vi "Add_to_speed_calib_file.vi"(2 "Desired Velocity":dbl format="%.2f", 3 "Max Velocity":dbl format="%.2f", 4 "New Row":dbl[](array[numeric]) format="%.2f", 6 "Rig Name":string, 7 "Mode":enum16{"Add Row", "Get Error Value"}(ring)) -> (0 "Tweaked Demand":dbl format="%.4f", 1 "Calib Tweak %":dbl format="%.4f")   [LabVIEW 2015]
uses:
  Anemometry/Anemometry Sub Vis/File/Setup_Filetype.ctl
  Anemometry/Anemometry Sub Vis/Controls/In_Range.ctl
panel:
  out "Array":dbl[][](array[numeric]) format="%.4f"
  out "Channel Values":string[][](array[string])
  # "Dem Vel       Calib Tweak   Meas Vel"
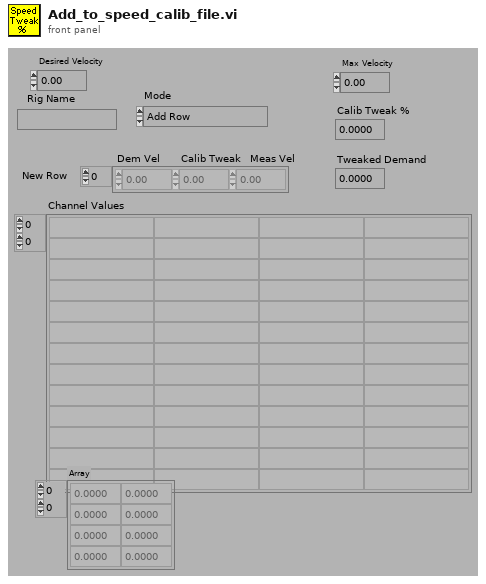
[diagram p1: front panel]
types:
  T1 = typedef "Setup_Filetype.ctl" = enum16{"Measurement Setups", "Calibration Setups", "General", "Results File Plotter Setups", "Speed Calib Tweaks"}
  T2 = typedef "In_Range.ctl" = enum16{"%", "±", "% & ±"}
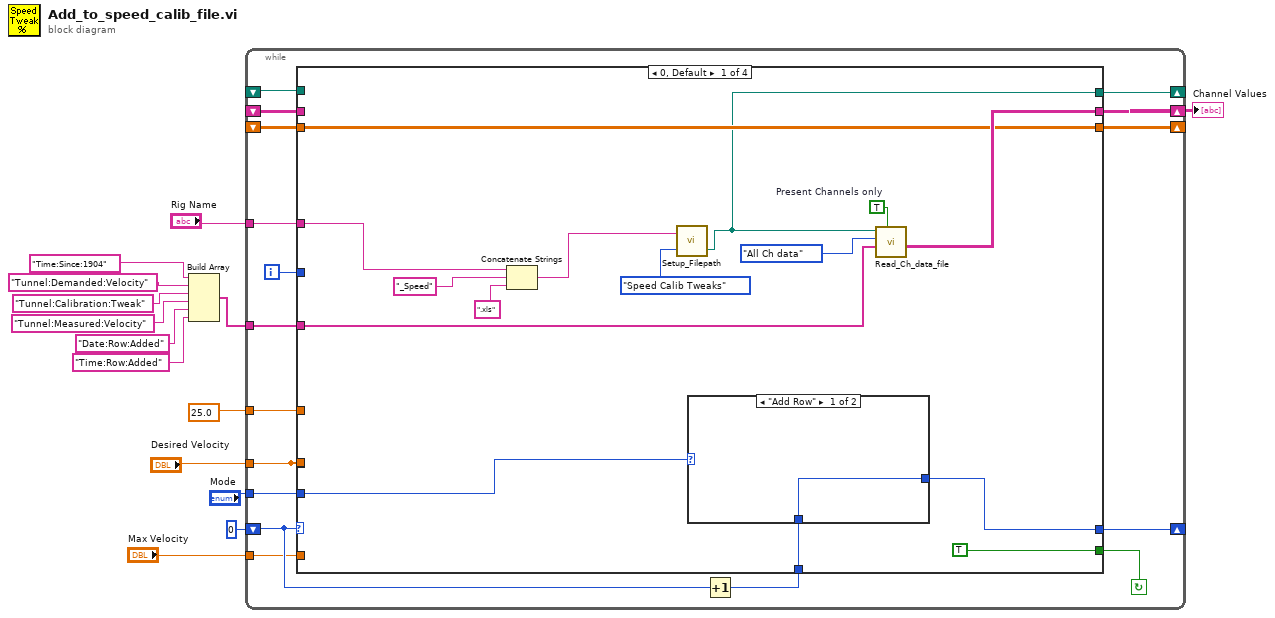
[diagram p0: block diagram]
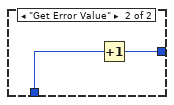
[diagram p2: hidden frame]
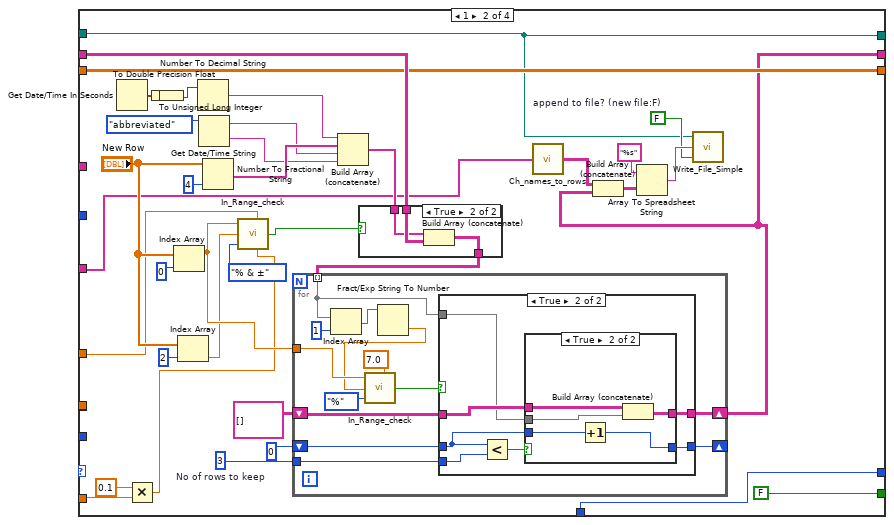
[diagram p3: hidden frame]
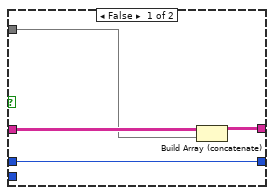
[diagram p5: hidden frame]
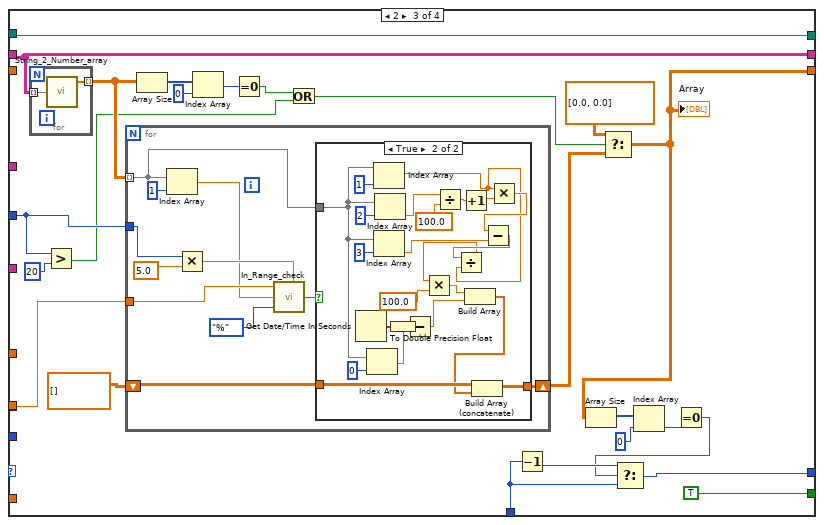
[diagram p7: hidden frame]
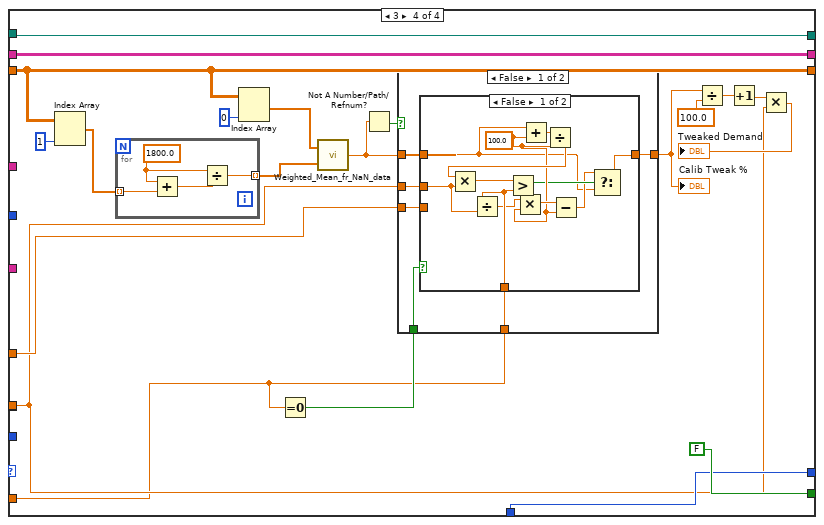
[diagram p9: hidden frame]
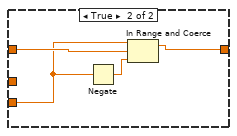
[diagram p10: hidden frame]
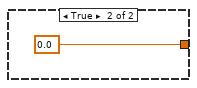
[diagram p11: hidden frame]
diagram:
  n1 = Build Array("Time:Since:1904" ("Substring"), "Tunnel:Demanded:Velocity" ("Substring"), "Tunnel:Calibration:Tweak" ("Substring"), "Tunnel:Measured:Velocity" ("Substring"), "Date:Row:Added" ("Substring"), "Time:Row:Added" ("Substring")) -> (w9:string[])
  n2 = while {
    tunnel: 25.0 ("Min") -> [w16]
    tunnel: "Desired Velocity" -> [w17]
    tunnel: "Rig Name" -> [w18]
    shift-left: _ -> [w19]
    shift-right: [w20] -> _
    tunnel: w9 -> [w26]
    shift-left: _ -> [w23]
    shift-right: [w24] -> w8
    shift-left: _ -> [w22]
    shift-right: [w25] -> _
    tunnel: "Mode" -> [w29]
    shift-left: 0 -> [w30]
    shift-right: [w28] -> _
    tunnel: "Max Velocity" -> [w15]
    i -> [w21]
    stop <- w31 continue-if-true
    n3 = Increment(x=w30) -> (x+1=w27:i32)
    n4 = case shown="0, Default" w30 {
      tunnel: [TRUE FALSE TRUE FALSE] -> w31
      tunnel: w29 -> [w44 _ _ _]
      tunnel: [w43 w76 w142 w198] -> w28
      tunnel: w27 -> [w42 w76 w144 w198]
      tunnel: w26 -> [w41 w55 _ _]
      tunnel: [w32 w56 w141 w203] -> w25
      tunnel: [w40 w54 w140 w202] -> w24
      tunnel: w23 -> [_ w82 w140 w202]
      tunnel: w22 -> [_ w56 w141 w203]
      tunnel: w21 -> [_ _ w129 _]
      tunnel: [w37 w80 w123 w186] -> w20
      tunnel: w19 -> [w37 w80 _ w186]
      tunnel: w18 -> [w36 _ _ _]
      tunnel: w17 -> [_ _ w133 _]
      tunnel: w17 -> [_ _ _ w185]
      tunnel: w16 -> [_ w50 _ w192]
      tunnel: w15 -> [_ w53 _ w183]
      frame 0, Default {
        w39 = TRUE  # Present Channels only
        n5 = Concatenate Strings(w36, "_Speed" ("Substring"), ".xls" ("string")) -> (w33:string)
        n6 = call "Setup_Filepath.vi"("Setup File Type"=Setup_Filetype."Speed Calib Tweaks", "Filename in"=w33) -> ("Filename Out"=w32:path)  [unwired: 1 out]
        n7 = case shown="\"Add Row\"" w44 {
          tunnel: [w47 w48] -> w43
          tunnel: w42 -> [w47 w49]
          frame "Add Row" {
          }
          frame "Get Error Value" {
            n8 = Increment(x=w49) -> (x+1=w48:i32)
          }
        }
        n9 = call "Read_Ch_data_file.vi"("Present Channels only"=w39, "Present Channels"=w41, "Output"=enum16{"All Ch data", "The last few rows"}."All Ch data", "Filename"=w32) -> ("Channel Values"=w40:string[][])  [unwired: 1 in, 4 out]
      }
      frame 1 {
        w57 = FALSE  # append to file? (new file:F)
        w74 = 3  # No of rows to keep
        n10 = Get Date/Time In Seconds() -> (seconds since 1Jan1904=w68:timestamp)
        n11 = Multiply(x=0.1, y=w53) -> (x*y=w51:dbl)
        n12 = To Double Precision Float(number=w68) -> (double precision float=w84:dbl)
        n13 = To Unsigned Long Integer(number=w84) -> (unsigned 32bit integer=w73:u32)
        n14 = Index Array(array="New Row", index=0 ("Index")) -> (element=w65:dbl)
        n15 = Index Array(array="New Row", index=2 ("Index")) -> (element=w64:dbl)
        n16 = Number To Decimal String(number=w73) -> (decimal integer string=w83:string)  [unwired: 1 out]
        n17 = Get Date/Time String(date format (0)=enum16{"short", "long", "abbreviated"}."abbreviated") -> (date string=w71:string, time string=w70:string)  [unwired: 2 out]
        n18 = Number To Fractional String(number="New Row", precision (6)=i16 4) -> (F-format string=w79:string[])  [unwired: 2 out]
        n19 = call "In_Range_check.vi"("±"=w51, "%"=w50, "Mode"=In_Range."% & ±", "Value"=w64, "Setpoint"=w65) -> ("In Range"=w62:bool)  [unwired: 2 out]
        n20 = Build Array (concatenate)(w83, w79, w71, w70) -> (w81:string[])
        n21 = case shown="True" w62 {
          tunnel: w82 -> [w87 w90]
          tunnel: w81 -> [_ w89]
          tunnel: [w87 w88] -> w78
          frame False {
          }
          frame True {
            n22 = Build Array (concatenate)(w89, w90) -> (w88:string[][])
          }
        }
        n23 = for {
          tunnel: w65 -> [w102]
          tunnel: w78 -> [w96] mode=indexing
          shift-right: [w94] -> w54
          shift-left: string[][] [] -> [w95]
          shift-right: [w93] -> _
          shift-left: 0 -> [w92]
          tunnel: w74 -> [w91]
          n24 = Index Array(array=w96, index=1 ("Index")) -> (element=w100:string)
          n25 = Fract/Exp String To Number(string=w100) -> (number=w99:dbl)  [unwired: 4 out]
          n26 = call "In_Range_check.vi"("%"=7.0, "Mode"=In_Range."%", "Value"=w99, "Setpoint"=w102) -> ("In Range"=w97:bool)  [unwired: 1 in, 2 out]
          n27 = case shown="True" w97 {
            tunnel: w96 -> [w106 w112]
            tunnel: w95 -> [w107 w113]
            tunnel: [w105 w111] -> w94
            tunnel: [w104 w109] -> w93
            tunnel: w92 -> [w104 w110]
            tunnel: w91 -> [_ w108]
            frame False {
              n28 = Build Array (concatenate)(w107, w106) -> (w105:string[][])
            }
            frame True {
              n29 = Less?(x=w110, y=w108) -> (x < y?=w114:bool)
              n30 = case shown="True" w114 {
                tunnel: w113 -> [w116 w121]
                tunnel: w112 -> [_ w120]
                tunnel: [w116 w119] -> w111
                tunnel: w110 -> [w115 w118]
                tunnel: [w115 w117] -> w109
                frame False {
                }
                frame True {
                  n31 = Increment(x=w118) -> (x+1=w117:i32)
                  n32 = Build Array (concatenate)(w121, w120) -> (w119:string[][])
                }
              }
            }
          }
        }
        n33 = call "Ch_names_to_rows.vi"("Channel Names"=w55) -> ("3 Row names"=w61:string[][])
        n34 = Build Array (concatenate)(w61, w54) -> (w59:string[][])
        n35 = Array To Spreadsheet String(array=w59, 3:"%s" ("format string")) -> (spreadsheet string=w58:string)  [unwired: 1 out]
        n36 = call "Write_File_Simple.vi"("append to file? (new file:F)"=w57, "character string"=w58, "file path"=w56) -> ()  [unwired: 2 out]
      }
      frame 2 {
        n37 = for {
          tunnel: w140 -> [w147] mode=indexing
          tunnel: [w146] -> w137 mode=indexing
          n38 = call "String_2_Number_array.vi"("Input String"=w147) -> ("Values"=w146:dbl[])
        }
        n39 = Greater?(x=w129, y=20) -> (0:w125:bool)
        n40 = for {
          tunnel: w137 -> [w152] mode=indexing
          tunnel: w129 -> [w149]
          tunnel: w133 -> [w157]
          shift-right: [w151] -> w124
          shift-left: dbl[][] [] -> [w153]
          n41 = Index Array(array=w152, index=1 ("Index")) -> (element=w148:dbl)
          n42 = Multiply(x=w149, y=5.0 ("x")) -> (x*y=w155:dbl)
          n43 = call "In_Range_check.vi"("%"=w155, "Mode"=In_Range."%", "Value"=w148, "Setpoint"=w157) -> ("In Range"=w154:bool)  [unwired: 1 in, 2 out]
          n44 = case shown="True" w154 {
            tunnel: w153 -> [w159 w182]
            tunnel: w152 -> [_ w168]
            tunnel: [w159 w181] -> w151
            frame False {
            }
            frame True {
              n45 = Get Date/Time In Seconds() -> (seconds since 1Jan1904=w166:timestamp)
              n46 = Index Array(array=w168, index=0 ("Index")) -> (element=w177:dbl)
              n47 = Index Array(array=w168, index=1 ("Index")) -> (element=w162:dbl)
              n48 = Index Array(array=w168, index=3 ("Index")) -> (element=w164:dbl)
              n49 = Index Array(array=w168, index=2 ("Index")) -> (element=w171:dbl)
              n50 = To Double Precision Float(number=w166) -> (double precision float=w178:dbl)
              n51 = Subtract(x=w178, y=w177) -> (x-y=w176:dbl)
              n52 = Divide(x=w171, y=100.0) -> (x/y=w172:dbl)
              n53 = Increment(x=w172) -> (x+1=w170:dbl)
              n54 = Multiply(x=w162, y=w170) -> (x*y=w165:dbl)
              n55 = Subtract(x=w165, y=w164) -> (x-y=w163:dbl)
              n56 = Divide(x=w163, y=w162) -> (x/y=w160:dbl)
              n57 = Multiply(x=w160, y=100.0) -> (x*y=w161:dbl)
              n58 = Build Array(w161, w176) -> (w175:dbl[])
              n59 = Build Array (concatenate)(w182, w175) -> (w181:dbl[][])
            }
          }
        }
        n60 = Array Size(array=w137) -> (size(s)=w136:i32[])
        n61 = Index Array(array=w136, index=0 ("Index")) -> (element=w134:i32)
        n62 = Equal To 0?(x=w134) -> (x = 0?=w127:bool)
        n63 = Or(x=w127, y=w125) -> (x .or. y?=w126:bool)
        n64 = Decrement(x=w144) -> (x-1=w143:i32)
        n65 = Select(t=dbl[][] [[0.0, 0.0]], s=w126, f=w124) -> (s? t:f=w123:dbl[][])
        "Array" <- w123
        n66 = Array Size(array=w123) -> (size(s)=w132:i32[])
        n67 = Index Array(array=w132, index=0 ("Index")) -> (element=w131:i32)
        n68 = Equal To 0?(x=w131) -> (x = 0?=w122:bool)
        n69 = Select(t=w143, s=w122, f=w144) -> (s? t:f=w142:i32)
      }
      frame 3 {
        n70 = Index Array(array=w186, index (col)=1 ("Index")) -> (element=w194:dbl[])  [unwired: 1 in]
        n71 = for {
          tunnel: w194 -> [w207] mode=indexing
          tunnel: [w204] -> w193 mode=indexing
          w205 = 1800.0
          n72 = Add(x=w205, y=w207) -> (x+y=w206:dbl)
          n73 = Divide(x=w205, y=w206) -> (x/y=w204:dbl)
        }
        n74 = Index Array(array=w186, index (col)=0 ("Index")) -> (element=w195:dbl[])  [unwired: 1 in]
        n75 = Equal To 0?(x=w183) -> (x = 0?=w184:bool)
        n76 = call "Weighted_Mean_fr_NaN_data.vi"("Weighting"=w193, "Data"=w195) -> ("Mean value"=w199:dbl)
        n77 = Not A Number/Path/Refnum?(number/path/refnum=w199) -> (NaN/Path/Refnum?=w200:bool)
        n78 = case shown="False" w200 {
          tunnel: w199 -> [w211 _]
          tunnel: [w210 0.0 ("Clamped output")] -> w191
          tunnel: w192 -> [w208 _]
          tunnel: w185 -> [w213 _]
          tunnel: w183 -> [w212 _]
          tunnel: w184 -> [w209 _]
          frame False {
            n79 = case shown="False" w209 {
              tunnel: w213 -> [w222 _]
              tunnel: w212 -> [w221 _]
              tunnel: w211 -> [w215 w229]
              tunnel: [w214 w226] -> w210
              tunnel: w208 -> [_ w228]
              frame False {
                w218 = 100.0 ("y")
                n80 = Divide(x=w221, y=w222) -> (x/y=w220:dbl)
                n81 = Multiply(x=w220, y=w218) -> (x*y=w219:dbl)
                n82 = Add(x=w215, y=w218) -> (x+y=w225:dbl)
                n83 = Divide(x=w225, y=w218) -> (x/y=w224:dbl)
                n84 = Multiply(x=w224, y=w222) -> (x*y=w223:dbl)
                n85 = Greater?(x=w223, y=w221) -> (0:w217:bool)
                n86 = Subtract(x=w219, y=w218) -> (x-y=w216:dbl)
                n87 = Select(t=w216, s=w217, f=w215) -> (s? t:f=w214:dbl)
              }
              frame True {
                n88 = Negate(x=w228) -> (-x=w227:dbl)
                n89 = In Range and Coerce(upper limit=w228, x=w229, lower limit=w227) -> (coerced(x)=w226:dbl)  [unwired: 1 out]
              }
            }
          }
          frame True {
          }
        }
        "Calib Tweak %" <- w191
        n90 = Divide(x=w191, y=100.0) -> (x/y=w189:dbl)
        n91 = Increment(x=w189) -> (x+1=w188:dbl)
        n92 = Multiply(x=w188, y=w185) -> (x*y=→"Tweaked Demand":dbl)
      }
    }
  }
  "Channel Values" <- w8
